vi "GDSAPI_Example_CreateNewProject.vi"(8 "error in (no error)":errorcluster, 10 "Base Folder(c:\\Temp\\GDS_Example)":path=path "c:/Temp/GDS_Example", 11 "NameOfLibrary(Ignored if empty)":string) -> (0 "error out":errorcluster, 2 "ProjectItem out":refnum<vi>, 3 "ProjectFolder":path, 5 "ProjectRefOut":refnum<vi>)   [LabVIEW 2014]
doc: "Helping VI to create a new project every time it's executed"
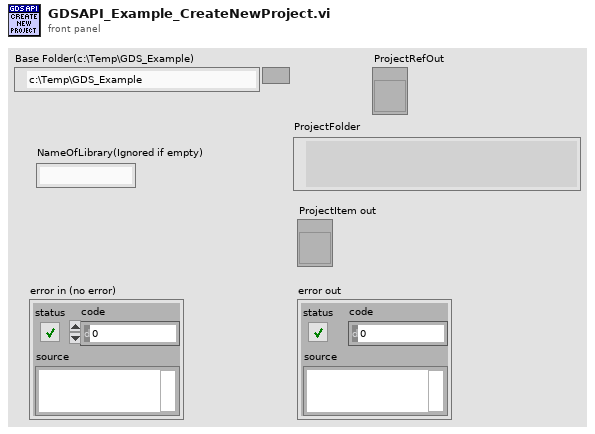
[diagram p1: front panel]
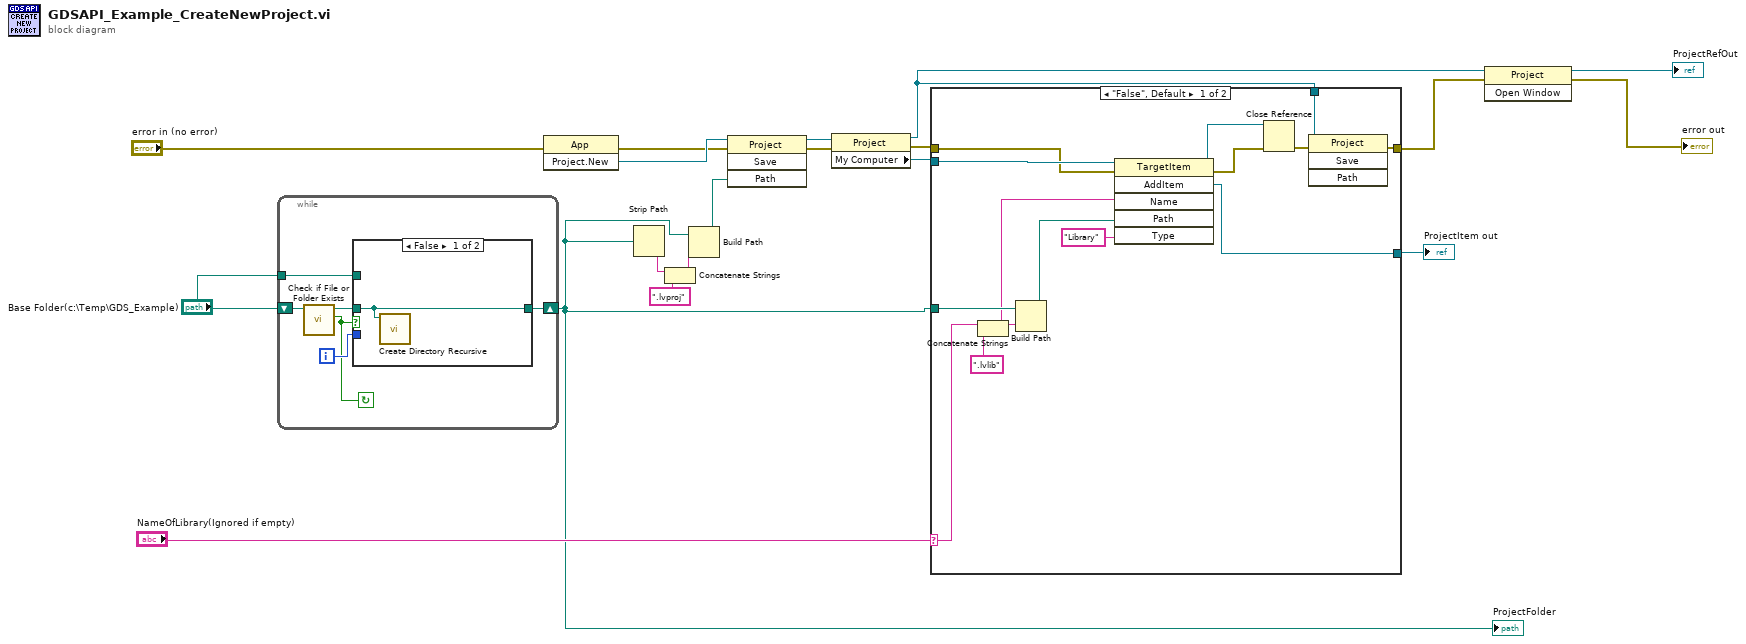
[diagram p0: block diagram]
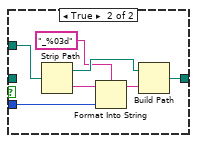
[diagram p3: hidden frame]
diagram:
  n1 = while {
    shift-right: [w23] -> w7
    shift-left: "Base Folder(c:\\Temp\\GDS_Example)" -> [w25]
    tunnel: "Base Folder(c:\\Temp\\GDS_Example)" -> [w21]
    i -> [w24]
    stop <- w22 continue-if-true
    n2 = call <vilib>:"Check if File or Folder Exists.vi"("path"=w25) -> ("file or folder exists?"=w22:bool, "dup path"=w20:path)  [unwired: 8 in, 1 out]
    n3 = case shown="False" w22 {
      tunnel: w21 -> [_ w33]
      tunnel: w24 -> [_ w31]
      tunnel: [w26 w27] -> w23
      tunnel: w20 -> [w26 _]
      frame False {
        n4 = call <vilib>:"Create Directory Recursive.vi"("directory"=w26) -> ()  [unwired: 4 in, 3 out]
      }
      frame True {
        n5 = Strip Path(path=w33) -> (stripped path=w32:path, name=w30:string)
        n6 = Format Into String(format string="_%03d", initial string=w30, w31) -> (resulting string=w28:string)  [unwired: 1 in, 1 out]
        n7 = Build Path(base path=w32, name or relative path=w28) -> (appended path=w27:path)
      }
    }
  }
  "ProjectFolder" <- w7
  n8 = invoke class="App" method="Project.New"(error in="error in (no error)") -> (error out=w17:errorcluster, "Project:New"=w18:refnum<vi>)  [unwired: 2 in, 1 out]
  n9 = Strip Path(path=w7) -> (name=w10:string)  [unwired: 1 out]
  n10 = Concatenate Strings(w10, ".lvproj" ("string")) -> (w8:string)
  n11 = Build Path(base path=w7, name or relative path=w8) -> (appended path=w11:path)
  n12 = invoke class="Project" method="Save"(reference=w18, error in=w17, "Path"=w11) -> (reference out=w15:refnum<vi>, error out=w16:errorcluster)  [unwired: 1 in, 2 out]
  n13 = property class="Project"(reference=w15, error in=w16) -> (reference out=w4:refnum<vi>, error out=w13:errorcluster, "My Computer"=w12:refnum<vi>)
  n14 = case shown="\"False\", Default" "NameOfLibrary(Ignored if empty)" {
    selector: "NameOfLibrary(Ignored if empty)" -> [w45 _]
    tunnel: w13 -> [w40 w49]
    tunnel: [w35 w49] -> w1
    tunnel: [w39 w48] -> w5
    tunnel: w12 -> [w47 w48]
    tunnel: w7 -> [w43 _]
    tunnel: w4 -> [w34 _]
    frame "False", Default {
      n15 = Concatenate Strings(w45, ".lvlib" ("string")) -> (w42:string)
      n16 = Build Path(base path=w43, name or relative path=w42) -> (appended path=w41:path)
      n17 = invoke class="TargetItem" method="AddItem"(reference=w47, error in=w40, "Name"=w42, "Path"=w41, "Type"="Library") -> (reference out=w37:refnum<vi>, error out=w38:errorcluster, "AddItem"=w39:refnum<vi>)  [unwired: 1 in, 3 out]
      n18 = Close Reference(reference=w37, error in (no error)=w38) -> (error out=w36:errorcluster)
      n19 = invoke class="Project" method="Save"(reference=w34, error in=w36) -> (error out=w35:errorcluster)  [unwired: 2 in, 3 out]
    }
    frame "" {
    }
  }
  "ProjectItem out" <- w5
  n20 = invoke class="Project" method="Open Window"(reference=w4, error in=w1) -> (reference out=→"ProjectRefOut":refnum<vi>, error out=→"error out":errorcluster)  [unwired: 1 in, 1 out]
